vi "AreaOfTriangle.vi"() -> ()   [LabVIEW 2024]
panel:
  out "Area":dbl
  in  "Height":dbl
  in  "Base":dbl
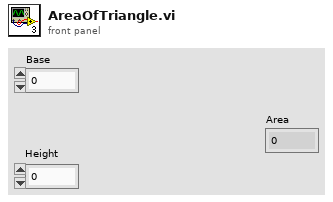
[diagram p1: front panel]
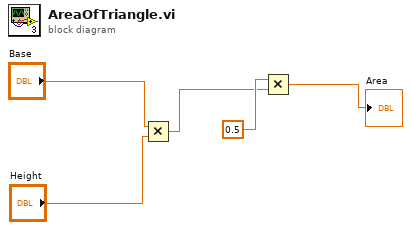
[diagram p0: block diagram]
diagram:
  n1 = Multiply(x="Base", y="Height") -> (x*y=w2:dbl)
  n2 = Multiply(x=0.5, y=w2) -> (x*y=→"Area":dbl)
